vi "get default data table.vi"(11 "data dictionary in":refnum<class "data bus dictionary.lvclass">) -> (2 "default data table":T1, 3 "data dictionary out":refnum<class "data bus dictionary.lvclass">)   [LabVIEW 2013, in "data bus dictionary.lvclass"]
doc: "Retrieves the default data table stored within the dictionary. This table is based on the default value provided by the tag descriptor during initialization."
uses:
  data bus dictionary.lvclass
  table/data table.ctl
  data bus dictionary.lvclass/data bus dictionary.ctl
  table/data bus values.lvlib
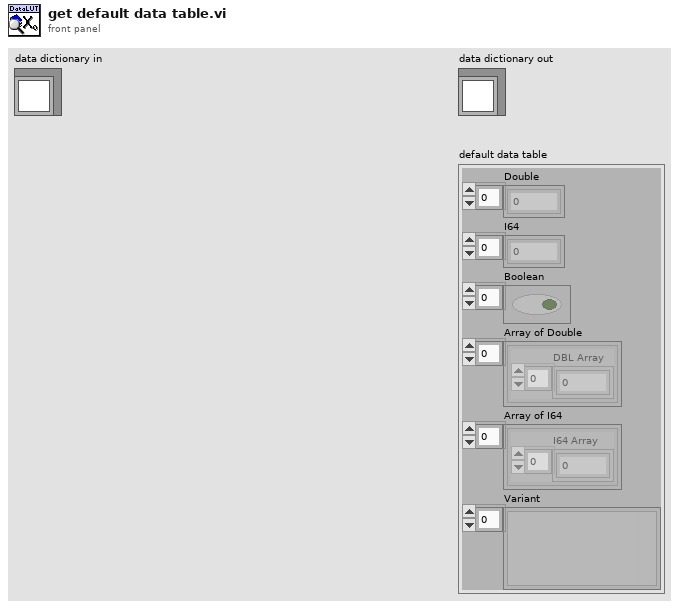
[diagram p1: front panel]
types:
  T1 = typedef "data bus values.lvlib/data table.ctl" = cluster{"Double":dbl[], "I64":i64[], "Boolean":bool[], "Array of Double":cluster{"DBL Array":dbl[]}[], "Array of I64":cluster{"I64 Array":i64[]}[], "Variant":variant[]}
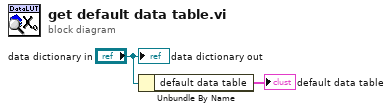
[diagram p0: block diagram]
diagram:
  n1 = Unbundle By Name("data dictionary in") -> ("default data table"=→"default data table":T1)
  "data dictionary out" <- "data dictionary in"
